vi "Configure Range Table (Harmonic Distortion).vi"(0 "VISA resource name":refnum<visa-resource-name>, 1 "Resolution Bandwidth":T3={"Enable Auto Resolution Bandwidth"=[TRUE, TRUE], "Manual Resolution Bandwidth"=[100000, 100000]}, 2 "Video Bandwidth":T2={"Enable Auto Video Bandwidth"=[FALSE, FALSE], "Manual Video Bandwidth"=[1000, 1000]}, 3 "Sweep Time":T1={"Enable Auto Sweep Time"=[TRUE, TRUE], "Sweep Time Value"=[0.01, 0.01]} {"Sweep Time Value" format="%#.6g"}, 5 "Range States":bool[](array[boolean])=[TRUE, TRUE], 7 "Center Frequency":dbl[](array[numeric])=[1000000000.0, 1000000000.0] format="%#.6g", 9 "Span":dbl[](array[numeric])=[0.0, 0.0], 11 "error in (no error)":errorcluster) -> (4 "VISA resource name out":refnum<visa-resource-name>, 15 "error out":errorcluster)   [LabVIEW 2014, in "Agilent ESA PSA Series.lvlib"]
doc: "Sets the frequency,bandwidth,sweep time for the specified range for spectrum analyzer Harmonic Distortion Measurement."
uses:
  Agilent ESA PSA Series.lvlib
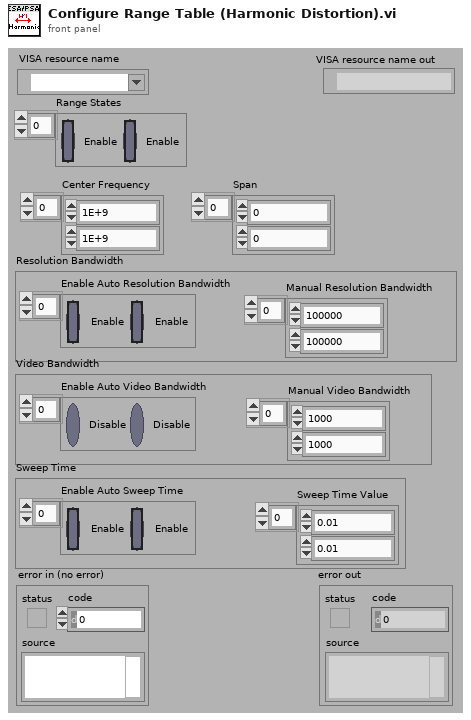
[diagram p1: front panel]
types:
  T1 = cluster{"Enable Auto Sweep Time":bool[], "Sweep Time Value":dbl[]}
  T2 = cluster{"Enable Auto Video Bandwidth":bool[], "Manual Video Bandwidth":i32[]}
  T3 = cluster{"Enable Auto Resolution Bandwidth":bool[], "Manual Resolution Bandwidth":i32[]}
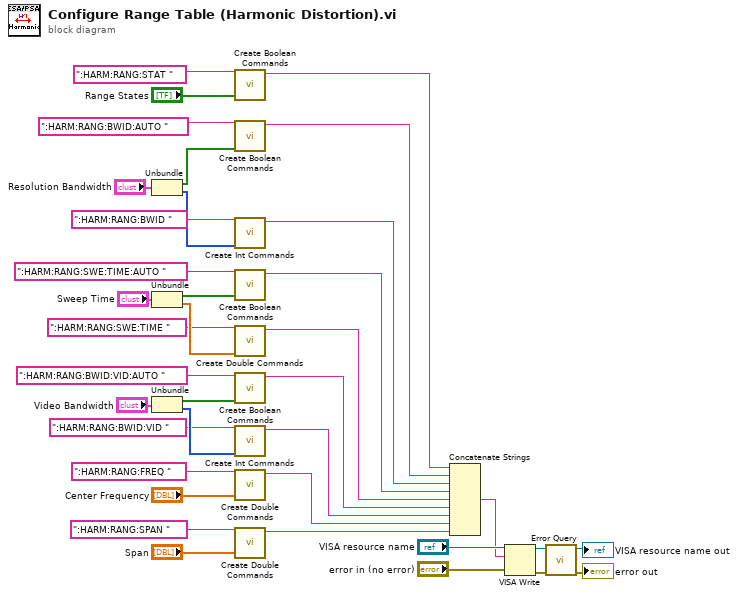
[diagram p0: block diagram]
diagram:
  n1 = Unbundle("Resolution Bandwidth") -> ("Enable Auto Resolution Bandwidth"=w23:bool[], "Manual Resolution Bandwidth"=w21:i32[])
  n2 = Unbundle("Sweep Time") -> ("Enable Auto Sweep Time"=w20:bool[], "Sweep Time Value"=w25:dbl[])
  n3 = Unbundle("Video Bandwidth") -> ("Enable Auto Video Bandwidth"=w17:bool[], "Manual Video Bandwidth"=w16:i32[])
  n4 = call "Create Boolean Commands.vi"("States"="Range States", "Command"=":HARM:RANG:STAT ") -> ("Result String"=w9:string)  [unwired: 9 in]
  n5 = call "Create Boolean Commands.vi"("States"=w23, "Command"=":HARM:RANG:BWID:AUTO ") -> ("Result String"=w8:string)  [unwired: 9 in]
  n6 = call "Create Int Commands.vi"("Values"=w21, "Commands"=":HARM:RANG:BWID ") -> ("Result"=w7:string)  [unwired: 9 in]
  n7 = call "Create Boolean Commands.vi"("States"=w20, "Command"=":HARM:RANG:SWE:TIME:AUTO ") -> ("Result String"=w6:string)  [unwired: 9 in]
  n8 = call "Create Double Commands.vi"("Double Values"=w25, "Commands"=":HARM:RANG:SWE:TIME ") -> ("Result"=w5:string)  [unwired: 9 in]
  n9 = call "Create Boolean Commands.vi"("States"=w17, "Command"=":HARM:RANG:BWID:VID:AUTO ") -> ("Result String"=w4:string)  [unwired: 9 in]
  n10 = call "Create Int Commands.vi"("Values"=w16, "Commands"=":HARM:RANG:BWID:VID ") -> ("Result"=w3:string)  [unwired: 9 in]
  n11 = call "Create Double Commands.vi"("Double Values"="Center Frequency", "Commands"=":HARM:RANG:FREQ ") -> ("Result"=w2:string)  [unwired: 9 in]
  n12 = call "Create Double Commands.vi"("Double Values"="Span", "Commands"=":HARM:RANG:SPAN ") -> ("Result"=w1:string)  [unwired: 9 in]
  n13 = Concatenate Strings(w9, w8, w7, w6, w5, w4, w3, w2, w1) -> (w28:string)
  n14 = VISA Write(VISA resource name="VISA resource name", write buffer=w28, error in (no error)="error in (no error)") -> (VISA resource name out=w34:refnum<visa-resource-name>, error out=w33:errorcluster)  [unwired: 1 out]
  n15 = call "Error Query.vi"("error in (no error)"=w33, "VISA resource name"=w34) -> ("error out"=→"error out":errorcluster, "VISA resource name out"=→"VISA resource name out":refnum<visa-resource-name>)  [unwired: 6 in, 2 out]
